vi "Main.vi"(11 "Module Admin":refnum<class "Delacor_lib_QMH_Cloneable Module Admin.lvclass">) -> ()   [LabVIEW 2018, in "CE14  Module.lvlib"]
doc: "This template is based off of the Queued Message Handler design pattern and the Queued Message Handler project template that ships with LabVIEW.\n\nThe main difference is that the queue is private to this module and communication between modules is performed via Broadcast and Request events.\n\nRequest events are wrapped in public API methods and are handled in the Event Handling Loop (EHL) of this VI. Any module can register for Broadcast events sent by this module. The EHL generates messages based on user interface actions.\n\nThe Message Handling Loop (MHL) processes messages generated by the EHL, or by other messages. The messages are string values, so new messages can be added easily to the Message Cases case structure in the MHL. Each message cluster can also provide an optional value for Message Data, which is a variant that can be converted to whatever message-specific data is required.\n_____\nBased on DQMH Project Template 6.0.0.91."
uses:
  CE14  Module.lvlib
  <vilib>/Delacor/Delacor QMH/Libraries/Cloneable Module Admin_class/Delacor_lib_QMH_Cloneable Module Admin.lvclass
  C:/Program Files (x86)/National Instruments/LabVIEW 2018/vi.lib/Delacor/Delacor QMH/Libraries/Module Admin_class/Delacor_lib_QMH_Module Admin.lvclass
  Module Data--cluster.ctl
  <vilib>/Delacor/Delacor QMH/Libraries/Message Queue_class/Delacor_lib_QMH_Message Queue.lvclass/Delacor_lib_QMH_Message Queue.ctl
  <vilib>/Delacor/Delacor QMH/Libraries/Cloneable Module Admin_class/Delacor_lib_QMH_Cloneable Module Admin.lvclass/Delacor_lib_QMH_Cloneable Module Admin.ctl
  Stop Argument--cluster.ctl
  <vilib>/Delacor/Delacor QMH/Libraries/Module Admin_class/Delacor_lib_QMH_Module Admin.lvclass/Delacor_lib_QMH_Module Admin.ctl
  Read AC para Argument--cluster.ctl
  <vilib>/Utility/miscctls.llb/LVPointTypeDef.ctl
  <vilib>/Delacor/Delacor QMH/Libraries/Message Queue_class/Delacor_lib_QMH_Enqueue Message (Single).vi
  <vilib>/Delacor/Delacor QMH/Libraries/Cloneable Module Admin_class/Delacor_lib_QMH_Get Module ID.vi
  <vilib>/Delacor/Delacor QMH/Libraries/Module Admin_class/Delacor_lib_QMH_Get External Launch.vi
  <vilib>/Utility/error.llb/Error Cluster From Error Code.vi
  <vilib>/ErrorRing/Error Ring.xnode
  <vilib>/Delacor/Delacor QMH/Libraries/Message Queue_class/Delacor_lib_QMH_Message Queue.lvclass
  Instrument Drivers/LVdriver_CE14(eMIC)/CE14_eMIC.lvlib
panel:
  in  "VISA resource name":refnum<visa-resource-name>
  out "error out":errorcluster
  out "Status":string
  in  "Simulate EHL Error":bool
  in  "Simulate MHL Error":bool
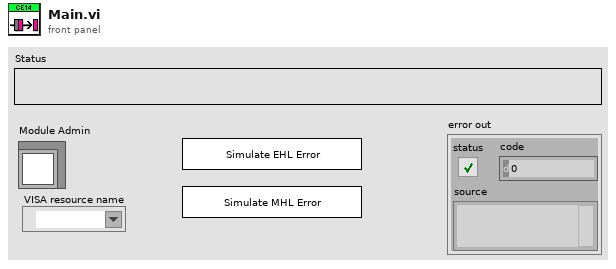
[diagram p1: front panel]
types:
  T1 = typedef "CE14  Module.lvlib/Request Events--cluster.ctl" = cluster{"Stop Module":refnum<user-event>, "Show Panel":refnum<user-event>, "Hide Panel":refnum<user-event>, "Show Diagram":refnum<user-event>, "Get Module Execution Status":refnum<user-event>, "Read AC para":refnum<user-event>}
  T2 = typedef "CE14  Module.lvlib/Module Data--cluster.ctl" = cluster{"Status":string, "VISA resource name":refnum<visa-resource-name>, "Success?":bool}
  T3 = enum32{"invalid lock state", "Not Locked", "Locked (No Password)", "Password-protected"}
  T4 = typedef "CE14  Module.lvlib/Stop Argument--cluster.ctl" = cluster{"Module ID":i32, "Origin":string, "Exit via Stop Module Req?":bool, "Wait for Module to stop?":bool}
  T5 = typedef "CE14  Module.lvlib/Read AC para Argument--cluster.ctl" = cluster{"Module ID":i32, "Boolean":bool}
  T6 = typedef "LVPointTypeDef.ctl" = cluster{"Horizontal":i16, "Vertical":i16}
  T7 = enum32{"Invalid", "Standard", "Closed", "Hidden", "Minimized", "Maximized"}
  T8 = typedef "CE14_eMIC.lvlib/CE14.data.ctl" = cluster{"strings":string, "float":dbl}
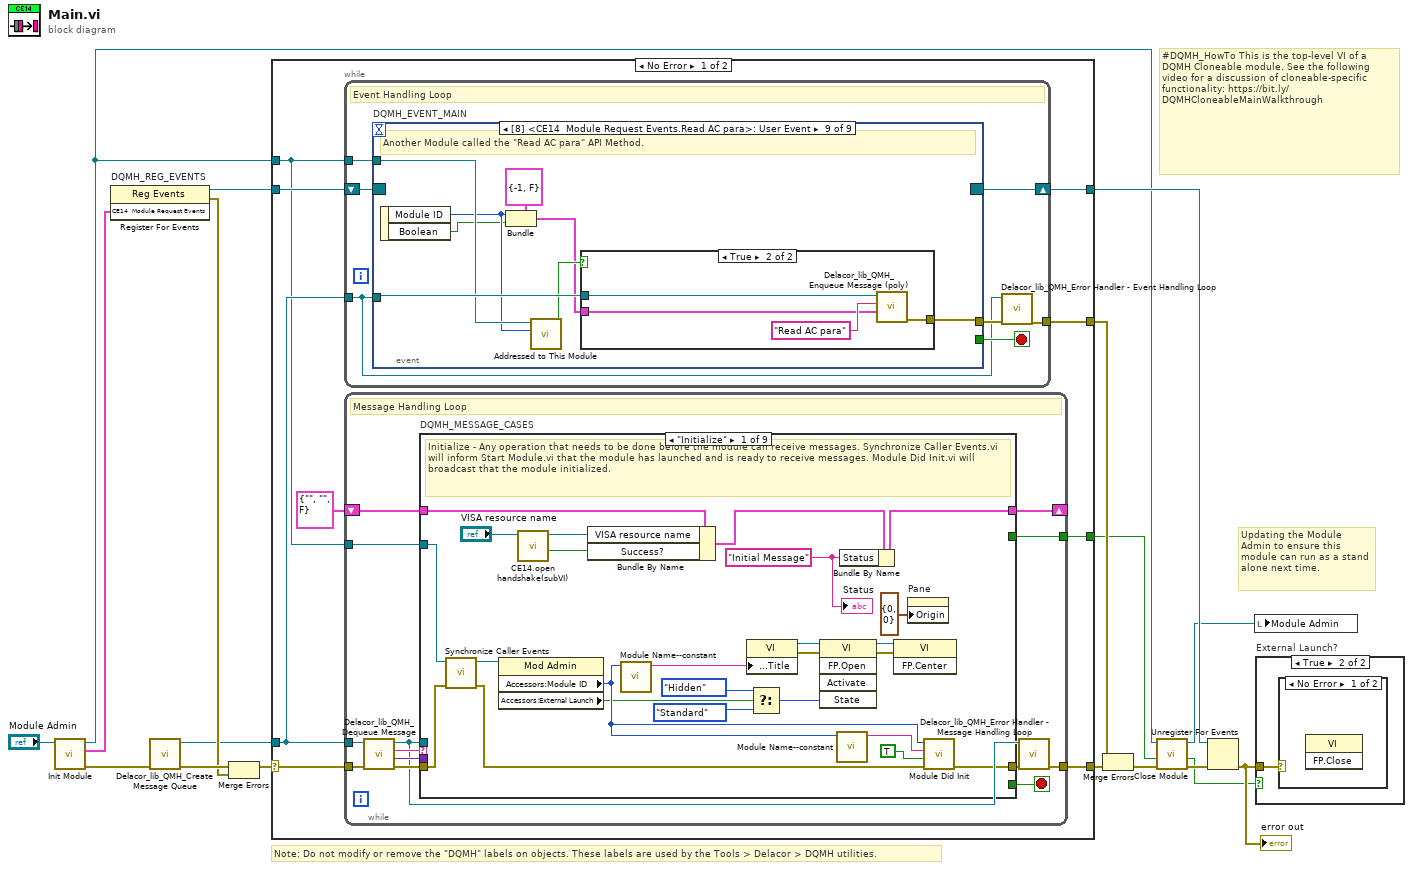
[diagram p0: block diagram]
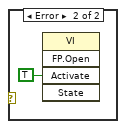
[diagram p3: hidden frame]
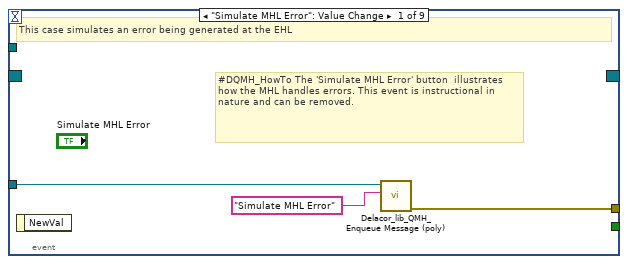
[diagram p4: hidden frame]
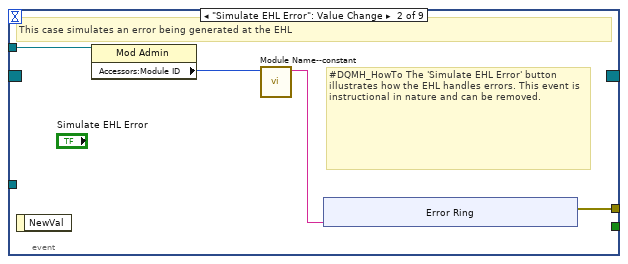
[diagram p5: hidden frame]
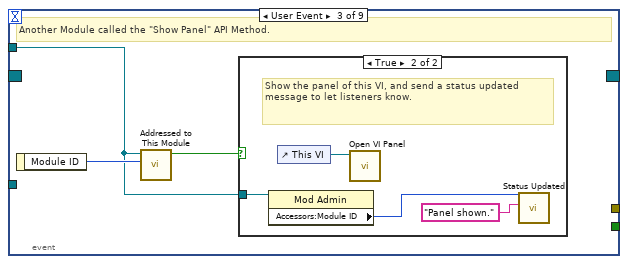
[diagram p6: hidden frame]
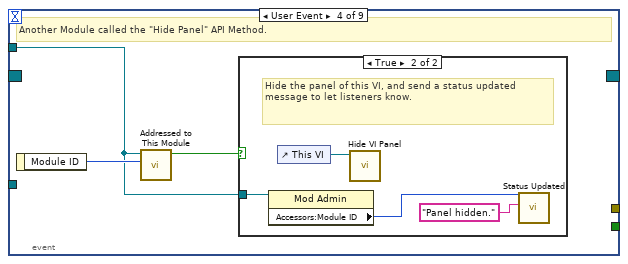
[diagram p8: hidden frame]
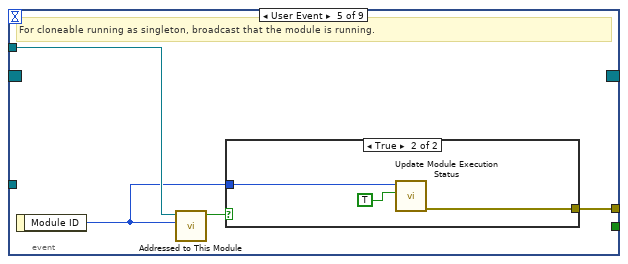
[diagram p10: hidden frame]
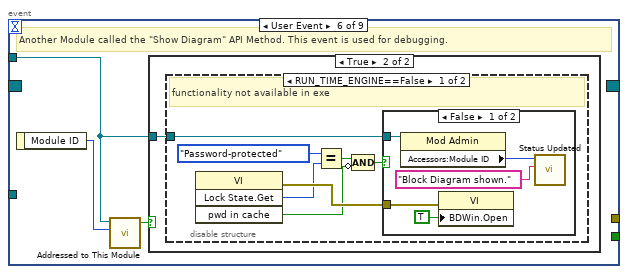
[diagram p12: hidden frame]
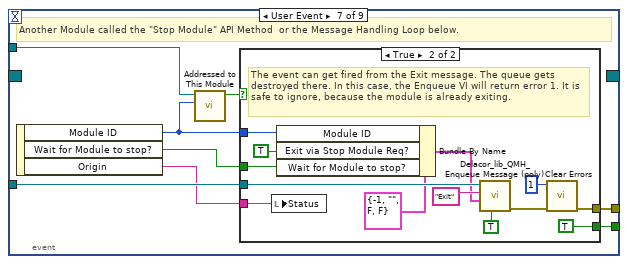
[diagram p16: hidden frame]
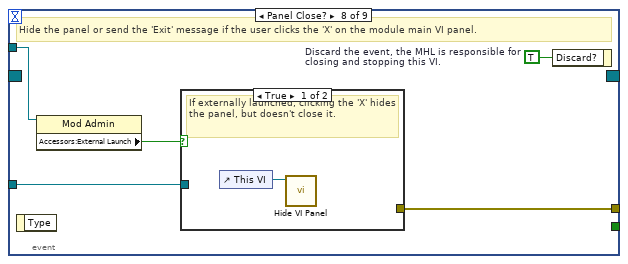
[diagram p18: hidden frame]
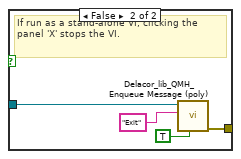
[diagram p19: hidden frame]
diagram:
  # "#DQMH_HowTo This is the top-level VI of a DQMH Cloneable module. See the following video for a discussion of cloneable-specific functionality: https://bit.ly/DQMHCloneableMainWalkthrough"
  # "Note: Do not modify or remove the \"DQMH\" labels on objects. These labels are used by the Tools > Delacor > DQMH utilities."
  # "Updating the Module Admin to ensure this module can run as a stand alone next time."
  n1 = call "Init Module.vi"("Cloneable Module Admin in"="Module Admin") -> ("error out"=w15:errorcluster, "CE14  Module Request Events"=w7:T1, "Cloneable Module Admin out"=w4:refnum<class "Delacor_lib_QMH_Cloneable Module Admin.lvclass">)  [unwired: 8 in]
  n2 = register-events "DQMH_REG_EVENTS"(w7) -> (reference out=w8:refnum<event-registration>, error out=w10:errorcluster)  [unwired: 2 in]
  n3 = call <vilib>:"Delacor_lib_QMH_Create Message Queue.vi"("error in"=w15) -> ("error out"=w12:errorcluster, "Message Queue"=w6:refnum<class "Delacor_lib_QMH_Message Queue.lvclass">)  [unwired: 9 in]
  n4 = Merge Errors(w12, w10) -> (w11:errorcluster)
  n5 = case shown="No Error" w11 {
    selector: w11 -> [w25 w266]
    tunnel: [w27 w265] -> w16
    tunnel: [w24 w273] -> w9
    tunnel: w8 -> [w22 w273]
    tunnel: w6 -> [w21 w264]
    tunnel: [w26 _] -> w17
    tunnel: w4 -> [w20 w269]
    tunnel: [w19 _] -> w2
    frame No Error {
      n6 = while {
        tunnel: w21 -> [w28]
        shift-right: [w31] -> w24
        shift-left: w22 -> [w32]
        tunnel: [w33] -> w26
        tunnel: w20 -> [w29]
        stop <- w30 stop-if-true
        # "Event Handling Loop"
        n7 = event "DQMH_EVENT_MAIN" shown="[8] <CE14  Module Request Events.Read AC para>: User Event" {
          selector: w32 -> [_ _ _ _ _ _ _ _ _]
          dyn-events: [_ _ _ _ _ _ _ _ _] -> w31
          timeout: _ -> [_ _ _ _ _ _ _ _ _]
          tunnel: [_ _ _ _ _ _ w89 _ _] -> w30
          tunnel: w28 -> [w36 _ _ _ _ _ w92 w108 w124]
          tunnel: [w37 w41 _ _ w66 _ w93 w111 w117] -> w34
          tunnel: w29 -> [_ w40 w49 w56 w64 w70 w91 w109 w122]
          event "Simulate MHL Error": Value Change {
            # "#DQMH_HowTo The 'Simulate MHL Error' button  illustrates how the MHL handles errors. This event is instructional in nature and can be removed."
            # "This case simulates an error being generated at the EHL"
            n8 = event-data() -> ()  [unwired: 1 in, 1 out]
            n9 = call-poly <vilib>:"Delacor_lib_QMH_Enqueue Message (poly).vi"("Message"="Simulate MHL Error", "Message Queue in"=w36) -> ("error out"=w37:errorcluster)  [unwired: 8 in, 1 out]
          }
          event "Simulate EHL Error": Value Change {
            # "#DQMH_HowTo The 'Simulate EHL Error' button  illustrates how the EHL handles errors. This event is instructional in nature and can be removed."
            # "This case simulates an error being generated at the EHL"
            n10 = event-data() -> ()  [unwired: 1 in, 1 out]
            n11 = property class="Mod Admin"(reference=w40) -> ("Accessors:Module ID"=w39:i32)  [unwired: 1 in, 2 out]
            n12 = call "Module Name--constant.vi"("Module ID"=w39) -> ("Module Name"=w38:string)  [unwired: 10 in]
            n13 = xnode "Error Ring"("parameter 0"=w38) -> ("error out"=w41:errorcluster)
          }
          event User Event {
            # "Another Module called the \"Show Panel\" API Method."
            n14 = event-data() -> ("Module ID"=w50:i32)  [unwired: 1 in]
            n15 = call "Addressed to This Module.vi"("Module ID from Argument"=w50, "Module Admin"=w49) -> ("Addressed to this instance?"=w51:bool)  [unwired: 8 in, 1 out]
            n16 = case shown="True" w51 {
              tunnel: w49 -> [_ w53]
              frame False {
              }
              frame True {
                # "Show the panel of this VI, and send a status updated message to let listeners know."
                n17 = property class="Mod Admin"(reference=w53) -> ("Accessors:Module ID"=w52:i32)  [unwired: 1 in, 2 out]
                n18 = control-ref of="This VI"() -> (w55:refnum<vi>)
                n19 = call "Open VI Panel.vi"("VI"=w55) -> ()  [unwired: 10 in, 1 out]
                n20 = call "Status Updated.vi"("Status"="Panel shown." ("format string"), "Module ID"=w52) -> ()  [unwired: 9 in, 1 out]
              }
            }
          }
          event User Event {
            # "Another Module called the \"Hide Panel\" API Method."
            n21 = event-data() -> ("Module ID"=w57:i32)  [unwired: 1 in]
            n22 = call "Addressed to This Module.vi"("Module ID from Argument"=w57, "Module Admin"=w56) -> ("Addressed to this instance?"=w58:bool)  [unwired: 8 in, 1 out]
            n23 = case shown="True" w58 {
              tunnel: w56 -> [_ w60]
              frame False {
              }
              frame True {
                # "Hide the panel of this VI, and send a status updated message to let listeners know."
                n24 = property class="Mod Admin"(reference=w60) -> ("Accessors:Module ID"=w59:i32)  [unwired: 1 in, 2 out]
                n25 = control-ref of="This VI"() -> (w62:refnum<vi>)
                n26 = call "Hide VI Panel.vi"("VI"=w62) -> ()  [unwired: 10 in, 1 out]
                n27 = call "Status Updated.vi"("Status"="Panel hidden." ("format string"), "Module ID"=w59) -> ()  [unwired: 9 in, 1 out]
              }
            }
          }
          event User Event {
            # "For cloneable running as singleton, broadcast that the module is running."
            n28 = event-data() -> ("Module ID"=w63:i32)  [unwired: 1 in]
            n29 = call "Addressed to This Module.vi"("Module ID from Argument"=w63, "Module Admin"=w64) -> ("Addressed to this instance?"=w65:bool)  [unwired: 8 in, 1 out]
            n30 = case shown="True" w65 {
              tunnel: [_ w69] -> w66
              tunnel: w63 -> [_ w68]
              frame False {
              }
              frame True {
                n31 = call "Update Module Execution Status.vi"("Running?"=TRUE, "Module ID"=w68) -> ("error out"=w69:errorcluster)  [unwired: 9 in]
              }
            }
          }
          event User Event {
            # "Another Module called the \"Show Diagram\" API Method. This event is used for debugging."
            n32 = event-data() -> ("Module ID"=w71:i32)  [unwired: 1 in]
            n33 = call "Addressed to This Module.vi"("Module ID from Argument"=w71, "Module Admin"=w70) -> ("Addressed to this instance?"=w72:bool)  [unwired: 8 in, 1 out]
            n34 = case shown="True" w72 {
              tunnel: w70 -> [_ w73]
              frame False {
              }
              frame True {
                n35 = disable-structure shown="RUN_TIME_ENGINE==False" {
                  disable-tunnel: w73 -> [w74 _]
                  frame condition #0 (active) {
                    # "functionality not available in exe"
                    n36 = invoke class="VI" method="Lock State.Get"() -> (error out=w80:errorcluster, "Get Lock State"=w79:T3, "pwd in cache"=w76:bool)  [unwired: 4 in, 1 out]
                    n37 = Equal?(x=T3."Password-protected", y=w79) -> (x = y?=w77:bool)
                    n38 = Compound Arithmetic op=AND(w77, invert w76) -> (w75:bool)
                    n39 = case shown="False" w75 {
                      tunnel: w80 -> [w85 _]
                      tunnel: w74 -> [w82 _]
                      frame False {
                        n40 = property class="Mod Admin"(reference=w82) -> ("Accessors:Module ID"=w81:i32)  [unwired: 1 in, 2 out]
                        n41 = property class="VI"(error in=w85, "BDWin.Open"=TRUE ("Block Diagram Window:Open")) -> ()  [unwired: 1 in, 2 out]
                        n42 = call "Status Updated.vi"("Status"="Block Diagram shown." ("format string"), "Module ID"=w81) -> ()  [unwired: 9 in, 1 out]
                      }
                      frame True {
                        # "Password-protected VI, and the password is not in the cache. Do not show the diagram."
                      }
                    }
                  }
                  frame condition #1 {
                  }
                }
              }
            }
          }
          event User Event {
            # "Another Module called the \"Stop Module\" API Method  or the Message Handling Loop below."
            n43 = event-data() -> ("Module ID"=w87:i32, "Wait for Module to stop?"=w88:bool, "Origin"=w86:string)  [unwired: 1 in]
            n44 = call "Addressed to This Module.vi"("Module ID from Argument"=w87, "Module Admin"=w91) -> ("Addressed to this instance?"=w90:bool)  [unwired: 8 in, 1 out]
            n45 = case shown="True" w90 {
              tunnel: [_ w105] -> w93
              tunnel: w92 -> [_ w101]
              tunnel: [_ TRUE] -> w89
              tunnel: w88 -> [_ w96]
              tunnel: w87 -> [_ w98]
              tunnel: w86 -> [_ w94]
              frame False {
              }
              frame True {
                # "The event can get fired from the Exit message. The queue gets destroyed there. In this case, the Enqueue VI will return error 1. It is safe to ignore, because the module is already exiting."
                n46 = local write "Status"(w94) -> ()
                n47 = Bundle By Name(cluster=T4 {"Module ID"=-1, "Origin"="", "Exit via Stop Module Req?"=FALSE, "Wait for Module to stop?"=FALSE} ("Stop Argument"), "Module ID"=w98, "Exit via Stop Module Req?"=TRUE, "Wait for Module to stop?"=w96) -> (w95:T4)
                n48 = call-poly <vilib>:"Delacor_lib_QMH_Enqueue Message (poly).vi"("Priority Message? (F)"=TRUE, "Message Data"=w95, "Message"="Exit", "Message Queue in"=w101) -> ("error out"=w106:errorcluster)  [unwired: 6 in, 1 out]
                n49 = call <vilib>:"Clear Errors.vi"("error in (no error)"=w106, "specific error code to clear (0: all)"=1) -> ("error out"=w105:errorcluster)  [unwired: 4 in, 1 out]
              }
            }
          }
          event Panel Close? {
            w110 = TRUE  # Discard the event, the MHL is responsible for closing and stopping this VI.
            # "Hide the panel or send the 'Exit' message if the user clicks the 'X' on the module main VI panel."
            n50 = event-data() -> ()  [unwired: 1 in, 1 out]
            n51 = property class="Mod Admin"(reference=w109) -> ("Accessors:External Launch"=w107:bool)  [unwired: 1 in, 2 out]
            n52 = case shown="True" w107 {
              tunnel: w108 -> [_ w115]
              tunnel: [_ w116] -> w111
              frame True {
                # "If externally launched, clicking the 'X' hides the panel, but doesn't close it."
                n53 = control-ref of="This VI"() -> (w112:refnum<vi>)
                n54 = call "Hide VI Panel.vi"("VI"=w112) -> ()  [unwired: 10 in, 1 out]
              }
              frame False {
                # "If run as a stand-alone VI, clicking the panel 'X' stops the VI."
                n55 = call-poly <vilib>:"Delacor_lib_QMH_Enqueue Message (poly).vi"("Priority Message? (F)"=TRUE, "Message"="Exit", "Message Queue in"=w115) -> ("error out"=w116:errorcluster)  [unwired: 7 in, 1 out]
              }
            }
            n56 = event-data("Discard?"=w110) -> ()  [unwired: 1 in, 1 out]
          }
          event User Event {
            # "Another Module called the \"Read AC para\" API Method."
            n57 = event-data() -> ("Module ID"=w119:i32, "Boolean"=w118:bool)  [unwired: 1 in]
            n58 = Bundle(cluster=T5 {"Module ID"=-1, "Boolean"=FALSE} ("Read AC para Argument"), "Module ID"=w119, "Boolean"=w118) -> (w120:T5)
            n59 = call "Addressed to This Module.vi"("Module ID from Argument"=w119, "Module Admin"=w122) -> ("Addressed to this instance?"=w123:bool)  [unwired: 8 in, 1 out]
            n60 = case shown="True" w123 {
              tunnel: w124 -> [_ w128]
              tunnel: w120 -> [_ w126]
              tunnel: [_ w125] -> w117
              frame False {
              }
              frame True {
                n61 = call-poly <vilib>:"Delacor_lib_QMH_Enqueue Message (poly).vi"("Message Data"=w126, "Message"="Read AC para", "Message Queue in"=w128) -> ("error out"=w125:errorcluster)  [unwired: 7 in, 1 out]
              }
            }
          }
        }
        n62 = call-dynamic "Delacor_lib_QMH_Error Handler - Event Handling Loop.vi"("error in"=w34, "Message Queue in"=w28) -> ("dup error in"=w33:errorcluster)  [unwired: 8 in, 1 out]
      }
      n63 = while {
        tunnel: w21 -> [w132]
        shift-right: [w136] -> _
        shift-left: T2 {"Status"="", "VISA resource name"="", "Success?"=FALSE} ("Data Cluster") -> [w137]
        tunnel: w25 -> [w140]
        tunnel: [w138] -> w27
        tunnel: w20 -> [w130]
        tunnel: [w129] -> w19
        stop <- w135 stop-if-true
        # "Message Handling Loop"
        n64 = call-dynamic "Delacor_lib_QMH_Dequeue Message.vi"("error in"=w140, "Message Queue in"=w132) -> ("error out"=w139:errorcluster, "Message Data"=w133:variant, "Message"=w134:string, "Message Queue out"=w131:refnum<class "Delacor_lib_QMH_Message Queue.lvclass">)  [unwired: 6 in]
        n65 = case "DQMH_MESSAGE_CASES" shown="\"Initialize\"" w134 {
          selector: w134 -> [_ _ _ _ _ _ _ _ w251]
          tunnel: w131 -> [_ _ _ _ _ w200 _ w241 _]
          tunnel: w139 -> [w164 w168 w193 w196 w198 w209 w222 w247 w253]
          tunnel: [w162 w168 w173 w195 w198 w205 w221 w244 w254] -> w141
          tunnel: w137 -> [w142 w167 w189 w194 w197 w204 w219 w232 w252]
          tunnel: [w155 w167 w189 w194 w197 w204 w219 w232 w252] -> w136
          tunnel: [_ _ _ _ _ _ _ w240 _] -> w135
          tunnel: w133 -> [_ _ w192 _ _ w203 _ w238 _]
          tunnel: w130 -> [w150 _ _ _ _ w202 w217 w234 w249]
          tunnel: [_ _ _ _ _ _ _ w236 _] -> w129
          frame "Initialize" {
            w147 = "Initial Message" ("Initial Message")
            # "Initialize - Any operation that needs to be done before the module can receive messages. Synchronize Caller Events.vi will inform Start Module.vi that the module has launched and is ready to receive messages. Module Did Init.vi will broadcast that the module initialized."
            n66 = call "Synchronize Caller Events.vi"("error in (no error)"=w164, "Module Admin"=w150) -> ("error out"=w163:errorcluster, "Module Admin out"=w149:refnum<class "Delacor_lib_QMH_Cloneable Module Admin.lvclass">)  [unwired: 8 in]
            n67 = property class="Mod Admin"(reference=w149) -> ("Accessors:Module ID"=w152:i32, "Accessors:External Launch"=w151:bool)  [unwired: 1 in, 2 out]
            n68 = call "CE14.open handshake(subVI).vi"("VISA resource name"="VISA resource name") -> ("success"=w145:bool, "VISA resource name 2"=w144:refnum<visa-resource-name>)  [unwired: 7 in, 2 out]
            n69 = Bundle By Name(cluster=w142, "VISA resource name"=w144, "Success?"=w145) -> (w143:T2)
            n70 = call "Module Name--constant.vi"("Module ID"=w152) -> ("Module Name"=w159:string)  [unwired: 10 in]
            n71 = property class="VI"("Front Panel.Title"=w159) -> (reference out=w161:refnum<vi>, error out=w166:errorcluster)  [unwired: 2 in]
            n72 = Select(t=T7."Hidden" ("State"), s=w151, f=T7."Standard" ("State")) -> (s? t:f=w156:T7)
            n73 = invoke class="VI" method="FP.Open"(reference=w161, error in=w166, "State"=w156) -> (reference out=w160:refnum<vi>, error out=w165:errorcluster)  [unwired: 2 in, 3 out]
            n74 = call "Module Name--constant.vi"("Module ID"=w152) -> ("Module Name"=w153:string)  [unwired: 10 in]
            n75 = Bundle By Name(cluster=w143, "Status"=w147) -> (w155:T2)
            n76 = invoke class="VI" method="FP.Center"(reference=w160, error in=w165) -> ()  [unwired: 1 in, 3 out]
            n77 = property on="Pane" class="Pane"("Origin"=T6 {"Horizontal"=0, "Vertical"=0}) -> ()  [unwired: 2 in, 2 out]
            n78 = call "Module Did Init.vi"("error in (no error)"=w163, "Initialized?"=TRUE, "Origin"=w153, "Module ID"=w152) -> ("error out"=w162:errorcluster)  [unwired: 7 in]
            "Status" <- w147
          }
          frame "---Module Specific---" {
            # "Separator -- The following cases handle messages specific to this Module."
          }
          frame "Read AC para" {
            # "Read ACV, ACI, PF, Freq, KW and broadcast when completed"
            n79 = Unbundle By Name(w189) -> ("VISA resource name"=w188:refnum<visa-resource-name>)
            n80 = Variant To Data(error in=w193, type=T5 {"Module ID"=-1, "Boolean"=FALSE} ("Read AC para Argument"), Variant=w192) -> (data=w190:T5, error out=w174:errorcluster)
            n81 = Unbundle By Name(w190) -> ("Module ID"=w171:i32)  [unwired: 1 out]
            n82 = call "CE14. Read_Voltage(subVI).vi"("VISA resource name"=w188) -> ("error out"=w183:errorcluster, "data out"=w179:T8, "VISA resource name out"=w187:refnum<visa-resource-name>)  [unwired: 7 in, 1 out]
            n83 = call "CE14. Read_Current(subVI).vi"("error in (no error)"=w183, "VISA resource name"=w187) -> ("error out"=w182:errorcluster, "data out"=w178:cluster{"strings":string, "float":dbl}, "VISA resource name out"=w186:refnum<visa-resource-name>)  [unwired: 6 in, 1 out]
            n84 = call "CE14. Read_Freq(subVI).vi"("error in (no error)"=w182, "VISA resource name"=w186) -> ("error out"=w181:errorcluster, "data out"=w177:T8, "VISA resource name out"=w185:refnum<visa-resource-name>)  [unwired: 6 in, 1 out]
            n85 = call "CE14. Read_PowerFactor(subVI).vi"("error in (no error)"=w181, "VISA resource name"=w185) -> ("error out"=w180:errorcluster, "data out"=w176:T8, "VISA resource name out"=w184:refnum<visa-resource-name>)  [unwired: 6 in, 1 out]
            n86 = call "CE14. Read_kW(subVI).vi"("error in (no error)"=w180, "VISA resource name"=w184) -> ("error out"=w172:errorcluster, "data out"=w175:T8)  [unwired: 6 in, 2 out]
            n87 = Build Array(w179, w178, w177, w176, w175) -> (w170:T8[])
            n88 = call "eMICs response.vi"("eMIC response"=w170, "Module ID"=w171) -> ("error out"=w169:errorcluster)  [unwired: 9 in]
            n89 = Merge Errors(w174, w172, w169) -> (w173:errorcluster)
          }
          frame "---Copy This Frame---" {
            # "Duplicate this frame when creating new messages.  Change this comment in the duplicated frame to describe this message."
            n90 = Merge Errors(w196) -> (w195:errorcluster)
          }
          frame "---Exit and Error Handling---" {
            # "Separator - the following cases handle errors and exit messages."
          }
          frame "Error" {
            # "#CodeRecommended - If you ever change the name of this \"Error\" message, you'll need to update the name in the Check Loop Error.vi as well."
            # "#CodeRecommended - If the module is running in standalone mode (External Launch = FALSE), this code will pop up an error dialog and call the 'Exit' message if an error occurs. Add more fine-grained error handling here."
            # "Error - Check the error message data and respond accordingly. This message is sent by the \"Error Handler\" VIs at the end of each loop in this application."
            n91 = property class="Mod Admin"(reference=w202) -> ("Accessors:External Launch"=w201:bool, "Accessors:Module ID"=w199:i32)  [unwired: 1 in, 2 out]
            n92 = Variant To Data(error in=w209, type=errorcluster {"status"=FALSE, "code"=0, "source"=""} ("error constant"), Variant=w203) -> (data=w210:errorcluster, error out=w207:errorcluster)
            n93 = call "Error Reported.vi"("Error"=w210, "Module ID"=w199) -> ()  [unwired: 9 in, 1 out]
            n94 = case shown="False" w201 {
              tunnel: [w215 _] -> w206
              tunnel: w200 -> [w213 _]
              tunnel: w210 -> [w214 _]
              frame False {
                # "If the module is running standalone, then pop up an error dialog and call the \"Exit\" message."
                n95 = call <vilib>:"Simple Error Handler.vi"("error in (no error)"=w214) -> ()  [unwired: 4 in, 5 out]
                n96 = call-poly <vilib>:"Delacor_lib_QMH_Enqueue Message (poly).vi"("Priority Message? (F)"=TRUE, "Message"="Exit", "Message Queue in"=w213) -> ("error out"=w215:errorcluster)  [unwired: 7 in, 1 out]
              }
              frame True {
                # "If the module was launched externally, calling the Error Reported broadcast VI is the only action performed by the \"Error\" message. The module's caller can then process the error appropriately."
              }
            }
            n97 = Merge Errors(w207, w206) -> (w205:errorcluster)
            n98 = local write "error out"(w205) -> ()
          }
          frame "Simulate MHL Error" {
            # "#DQMH_HowTo The 'Simulate MHL Error' button  illustrates how the MHL handles errors. This event is instructional in nature and can be removed."
            # "Simulate an error occurring at the MHL"
            n99 = property class="Mod Admin"(reference=w217) -> ("Accessors:Module ID"=w218:i32)  [unwired: 1 in, 2 out]
            n100 = call "Module Name--constant.vi"("Module ID"=w218) -> ("Module Name"=w216:string)  [unwired: 10 in]
            n101 = xnode "Error Ring"("parameter 0"=w216) -> ("error out"=w220:errorcluster)
            n102 = Merge Errors(w222, w220) -> (w221:errorcluster)
          }
          frame "Exit" {
            w239 = 91  # 91: not all Exit messages will have an argument
            w240 = TRUE  # Stop the VI
            # "Release the message queue reference"
            # "Exit - Exit the application."
            n103 = Variant To Data(error in=w247, type=T4 {"Module ID"=-1, "Origin"="", "Exit via Stop Module Req?"=FALSE, "Wait for Module to stop?"=FALSE} ("Stop Argument"), Variant=w238) -> (data=w235:T4, error out=w242:errorcluster)
            n104 = Unbundle By Name(w232) -> ("VISA resource name"=w231:refnum<visa-resource-name>)
            n105 = call <vilib>:"Clear Errors.vi"("error in (no error)"=w242, "specific error code to clear (0: all)"=w239) -> ("error out"=w246:errorcluster)  [unwired: 4 in, 1 out]
            n106 = control-ref of="This VI"() -> (w233:refnum<vi>)
            n107 = call "CE14 Close Connection (SubVI).vi"("VISA Refnum in"=w231) -> ("error out"=w230:errorcluster)  [unwired: 10 in]
            n108 = call-dynamic "Delacor_lib_QMH_Release Message Queue.vi"("error in"=w246, "Message Queue"=w241) -> ("error out"=w245:errorcluster)  [unwired: 9 in]
            n109 = call "Handle Exit.vi"("Stop Argument"=w235, "Module Admin in"=w234, "VI reference"=w233) -> ("error out"=w243:errorcluster, "Wait for Stop?"=w236:bool)  [unwired: 7 in]
            n110 = Merge Errors(w245, w243, w230) -> (w244:errorcluster)
          }
          frame Default {
            # "'Default' case only runs if there is a message that isn't defined in any of the other cases.  Output a programming error."
            n111 = property class="Mod Admin"(reference=w249) -> ("Accessors:Module ID"=w248:i32)  [unwired: 1 in, 2 out]
            n112 = call "Module Name--constant.vi"("Module ID"=w248) -> ("Module Name"=w250:string)  [unwired: 10 in]
            n113 = xnode "Error Ring"("parameter 0"=w251, "parameter 1"=w250) -> ("error out"=w255:errorcluster)
            n114 = Merge Errors(w253, w255) -> (w254:errorcluster)
          }
        }
        n115 = call-dynamic "Delacor_lib_QMH_Error Handler - Message Handling Loop.vi"("error in"=w141, "Message Queue in"=w131) -> ("dup error in"=w138:errorcluster)  [unwired: 8 in, 1 out]
      }
    }
    frame Error {
      n116 = call "Synchronize Caller Events.vi"("Module Admin"=w269) -> ("Module Admin out"=w268:refnum<class "Delacor_lib_QMH_Cloneable Module Admin.lvclass">)  [unwired: 9 in, 1 out]
      n117 = property class="Mod Admin"(reference=w268) -> ("Accessors:Module ID"=w267:i32)  [unwired: 1 in, 2 out]
      n118 = call-dynamic "Delacor_lib_QMH_Release Message Queue.vi"("error in"=w266, "Message Queue"=w264) -> ("error out"=w265:errorcluster)  [unwired: 9 in]
      n119 = call "Module Name--constant.vi"("Module ID"=w267) -> ("Module Name"=w272:string)  [unwired: 10 in]
      n120 = Format Into String(format string="An error occurred during initialization. %s is no longer running.", w272) -> (resulting string=w270:string)  [unwired: 2 in, 1 out]
      n121 = call "Error Reported.vi"("Additional Information"=w270, "Error"=w265, "Module ID"=w267) -> ()  [unwired: 8 in, 1 out]
    }
  }
  n122 = Merge Errors(w17, w16) -> (w18:errorcluster)
  n123 = call "Close Module.vi"("error in"=w18, "Wait for stop?"=w2, "Module Admin in"=w4) -> ("error out"=w14:errorcluster, "External Launch"=w1:bool, "Module Admin out"=w3:refnum<class "Delacor_lib_QMH_Cloneable Module Admin.lvclass">)  [unwired: 6 in]
  n124 = Unregister For Events(event registration refnum=w9, error in=w14) -> (error out=w13:errorcluster)
  "error out" <- w13
  n125 = local write "Module Admin"(w3) -> ()
  n126 = case "External Launch?" shown="True" w1 {
    tunnel: w13 -> [_ w274]
    frame False {
    }
    frame True {
      n127 = case shown="No Error" w274 {
        frame No Error {
          n128 = invoke class="VI" method="FP.Close"() -> ()  [unwired: 3 in, 3 out]
        }
        frame Error {
          n129 = invoke class="VI" method="FP.Open"("Activate"=TRUE ("Activate?")) -> ()  [unwired: 4 in, 5 out]
        }
      }
    }
  }
